vi "Write.vi"(8 "error in (no error)":errorcluster caption="entrée d'erreur (pas d'erreur)", 11 "Class CSV_File (Default) en entrée":refnum<class "Class File (Default).lvclass">) -> (0 "error out":errorcluster caption="sortie d'erreur", 3 "Class CSV_File (Default) en sortie":refnum<class "Class File (Default).lvclass">)   [LabVIEW 2020, in "Library Instrument & Equipement.lvlib" / "Library File.lvlib" / "Class File (Default).lvclass"]
uses:
  Class File (Default).lvclass
  Class File (Default).lvclass/Class File (Default).ctl
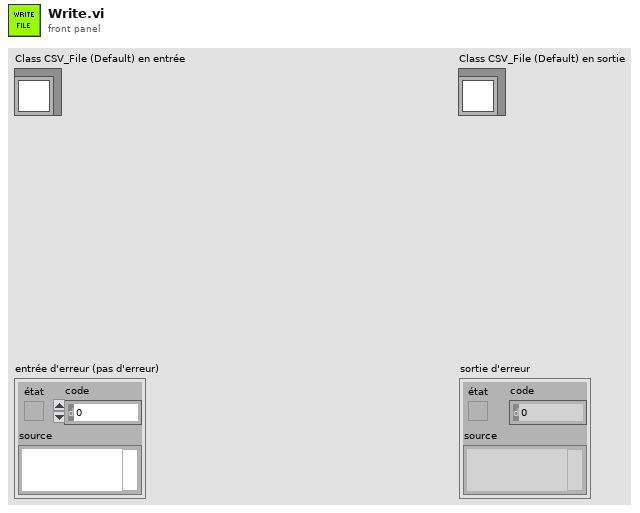
[diagram p1: front panel]
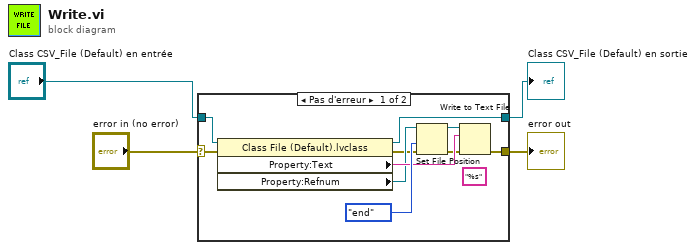
[diagram p0: block diagram]
diagram:
  n1 = case shown="Pas d'erreur" "error in (no error)" {
    selector: "error in (no error)" -> [w7 w16]
    tunnel: [w12 w16] -> w3
    tunnel: [w13 w15] -> w1
    tunnel: "Class CSV_File (Default) en entrée" -> [w14 w15]
    frame No Error {
      (unwired) "%s" ("chaîne de format")
      n2 = property class="Class File (Default).lvclass"(reference=w14, error in=w7) -> (reference out=w13:refnum<class "Class File (Default).lvclass">, error out=w6:errorcluster, "Property:Text"=w9:string, "Property:Refnum"=w8:refnum<file>)
      n3 = Set File Position(refnum=w8, from (0:start)=enum16{"start", "end", "current"}."end" ("à partir de (0 : start)"), error in=w6) -> (refnum out=w11:refnum<file>, error out=w5:errorcluster)  [unwired: 1 in]
      n4 = Write to Text File(file (use dialog)=w11, text=w9, error in=w5) -> (error out=w12:errorcluster)  [unwired: 1 in, 2 out]
    }
    frame Error {
    }
  }
  "error out" <- w3
  "Class CSV_File (Default) en sortie" <- w1
